vi "connect.vi"(8 "error in (no error)":errorcluster, 11 "TCPServer in":refnum<class "TCPServer.lvclass">) -> (0 "error out":errorcluster, 3 "TCPServer out":refnum<class "TCPServer.lvclass">)   [LabVIEW 2016, in "TCPServer.lvclass"]
uses:
  TCPServer.lvclass
  C:/Users/aanania/Documents/ss_atdome/ts_labview_tcp/TCPCommunicator/TCPCommunicator.lvclass
  TCPSettings/TCPSettings.lvclass/TCPSettings.ctl
  TCPCommunicator/TCPCommunicator.lvclass/TCPCommunicator.ctl
  TCPSettings/TCPSettings.lvclass
  TCPCommunicator/TCPCommunicator.lvclass
panel:
  out "port":u16
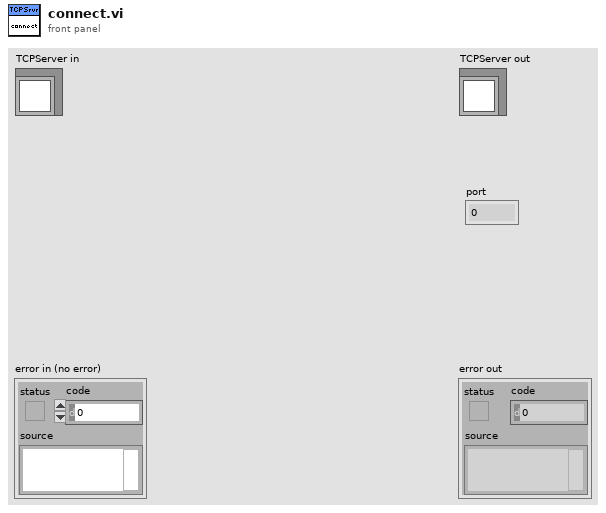
[diagram p1: front panel]
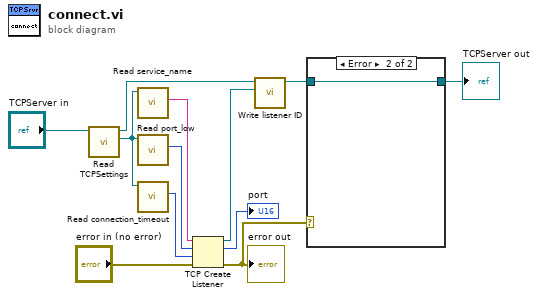
[diagram p0: block diagram]
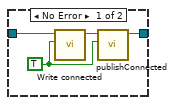
[diagram p2: hidden frame]
diagram:
  n1 = call-dynamic "Read TCPSettings.vi"("TCPCommunicator in"="TCPServer in") -> ("TCPSettings.lvclass"=w9:refnum<class "TCPSettings.lvclass">, "TCPCommunicator out"=w4:refnum<class "TCPServer.lvclass">)  [unwired: 8 in, 1 out]
  n2 = call "Read service_name.vi"("TCPSettings in"=w9) -> ("service_name"=w11:string)  [unwired: 8 in, 2 out]
  n3 = call-dynamic "Read port_low.vi"("TCPSettings in"=w9) -> ("port_low"=w12:u16)  [unwired: 8 in, 2 out]
  n4 = call-dynamic "Read connection_timeout .vi"("TCPSettings in"=w9) -> ("connection_timeout"=w10:i32)  [unwired: 8 in, 2 out]
  n5 = TCP Create Listener(8:"error in (no error)", 9:w10, 10:w12, 11:w11) -> (0:w1:errorcluster, 2:→"port":u16, 3:w3:refnum<k5>)  [unwired: 1 out]
  "error out" <- w1
  n6 = call "Write listener ID.vi"("listener ID"=w3, "TCPCommunicator in"=w4) -> ("TCPCommunicator out"=w5:refnum<class "TCPServer.lvclass">)  [unwired: 8 in, 1 out]
  n7 = case shown="Error" w1 {
    tunnel: w5 -> [w16 w17]
    tunnel: [w13 w17] -> w2
    frame No Error {
      w15 = TRUE ("connected")
      n8 = call "Write connected.vi"("connected"=w15, "TCPCommunicator in"=w16) -> ("TCPCommunicator out"=w14:refnum<class "TCPServer.lvclass">)  [unwired: 8 in, 1 out]
      n9 = call-dynamic "publishConnected.vi"("Connected"=w15, "TCPCommunicator in"=w14) -> ("TCPCommunicator out"=w13:refnum<class "TCPServer.lvclass">)  [unwired: 8 in, 1 out]
    }
    frame Error {
    }
  }
  "TCPServer out" <- w2
